vi "InitDone.vi"(8 "error in (no error)":errorcluster, 10 "Variant":variant, 11 "Arduino_TranslationStage_UI.lvlib:Arduino_Stepper.lvclass":refnum<class "Arduino_Stepper_UI.lvclass">) -> (0 "error out":errorcluster, 3 "Arduino_TranslationStage_UI.lvlib:Arduino_Stepper.lvclass":refnum<class "Arduino_Stepper_UI.lvclass">)   [LabVIEW 2023, in "Arduino_TranslationStage_UI.lvlib" / "Arduino_Stepper_UI.lvclass"]
uses:
  Arduino_Stepper_UI.lvclass
  Arduino_Stepper_UI.lvclass/Arduino_Stepper_UI.ctl
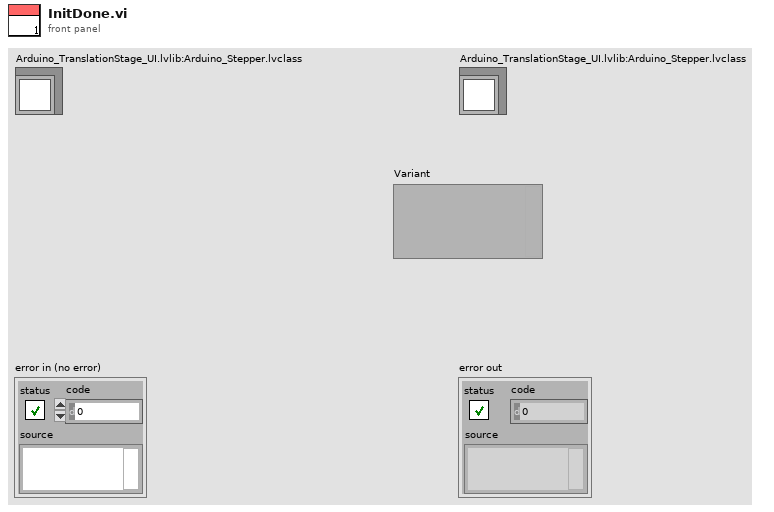
[diagram p1: front panel]
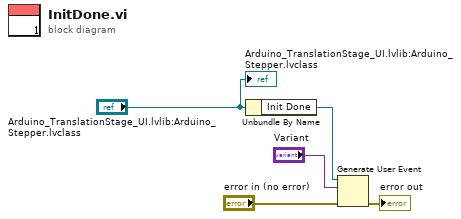
[diagram p0: block diagram]
diagram:
  n1 = Unbundle By Name("Arduino_TranslationStage_UI.lvlib:Arduino_Stepper.lvclass") -> ("Init Done"=w3:refnum<user-event>)
  n2 = Generate User Event(user event=w3, event data cluster="Variant", error in="error in (no error)") -> (error out=→"error out":errorcluster)  [unwired: 1 in, 1 out]
  "Arduino_TranslationStage_UI.lvlib:Arduino_Stepper.lvclass" <- "Arduino_TranslationStage_UI.lvlib:Arduino_Stepper.lvclass"
